vi "Check Watchdogs.vi"(7 "Check Period (ms)":u32=100, 8 "error in (no error)":errorcluster, 11 "RT - Analysis Data in in in in":T1={"Accel Sensistivity"=[0.0, 0.0, 0.0], "Cutoff Frequncies"=[{"LP Passband"=0.0, "HP Stopband"=0.0, "LP Stopband"=0.0, "HP Passband"=0.0}, {"LP Passband"=0.0, "HP Stopband"=0.0, "LP Stopband"=0.0, "HP Passband"=0.0}, {"LP Passband"=0.0, "HP Stopband"=0.0, "LP Stopband"=0.0, "HP Passband"=0.0}], "APU Setup File"={"Sensor Info"=[], "Calibration Info"=[], "CMM Table 106"=[], "CMM Table 106B "=[], "Accel Config"=[], "Report Sheet 1"=[], "Report Sheet 2"=[], "Report Sheet 3"=[]}, "RepairLevel"=""} {"Cutoff Frequncies"."HP Passband" min=1.0 step=1.0 format="%#.4f"; "Cutoff Frequncies"."LP Stopband" min=1.0 step=1.0 format="%#.4f"; "Cutoff Frequncies"."HP Stopband" min=1.0 step=1.0 format="%#.4f"; "Cutoff Frequncies"."LP Passband" min=1.0 step=1.0 format="%#.4f"}) -> (0 "error out":errorcluster, 3 "RT - Analysis Data in in out":T1 {"Cutoff Frequncies"."HP Passband" min=1.0 step=1.0 format="%#.4f"; "Cutoff Frequncies"."LP Stopband" min=1.0 step=1.0 format="%#.4f"; "Cutoff Frequncies"."HP Stopband" min=1.0 step=1.0 format="%#.4f"; "Cutoff Frequncies"."LP Passband" min=1.0 step=1.0 format="%#.4f"})   [LabVIEW 2018, in "RT - Analysis.lvlib"]
doc: "Runs through each Watchdog setting and checks for triggers.\n\n<b>Timer - Change Sample Rate</b>\nDBL0 : Timer Length\nDBL1 : New Sample Ratea\n\n<b>RPM Thresh - Insert Other</b> (Inserts Watchdog from variant)\nBool0 : T/F : RPMGreaterThan/RPMLessThan\nDBL0 : RPM Thresh Val\nVariant : Watchdog Cluster\n\n<b>RPM Thresh - Check POPD</b>\nBool0 : T/F : RPMGreaterThan/RPMLessThan\nBool1 : T/F : POPDGreaterThan/POPDLessThan\nDBL0 : RPM Thresh Val\nDBL1 : POPD Thresh Val\n\n<b>RPM Thresh - StartStop Logging</b>\nBool0 : T/F : RPMGreaterThan/RPMLessThan\nBool1 : T/F : StartLogg/FalseLogg\nDBL0 : Thresh Val"
uses:
  RT - Analysis.lvlib
  RT - Host Comms/RT - Host Comms.lvlib
  Public Controls/Alert Data.ctl
  Private Controls/Watchdog Settings.ctl
  Private Controls/RT-Analysis Data.ctl
  Modules/Testing UI 3/Private Controls/Cutoff Frequency.ctl
  Modules/Testing UI 3/Testing UI 3.lvlib
  Top Level/Shared Controls/APU Setup File.ctl
panel:
  # "Highpass Cutoff Frequency"
  # "Lowpass Cutoff Frequency"
  # "Highpass Cutoff Frequency"
  # "Lowpass Cutoff Frequency"
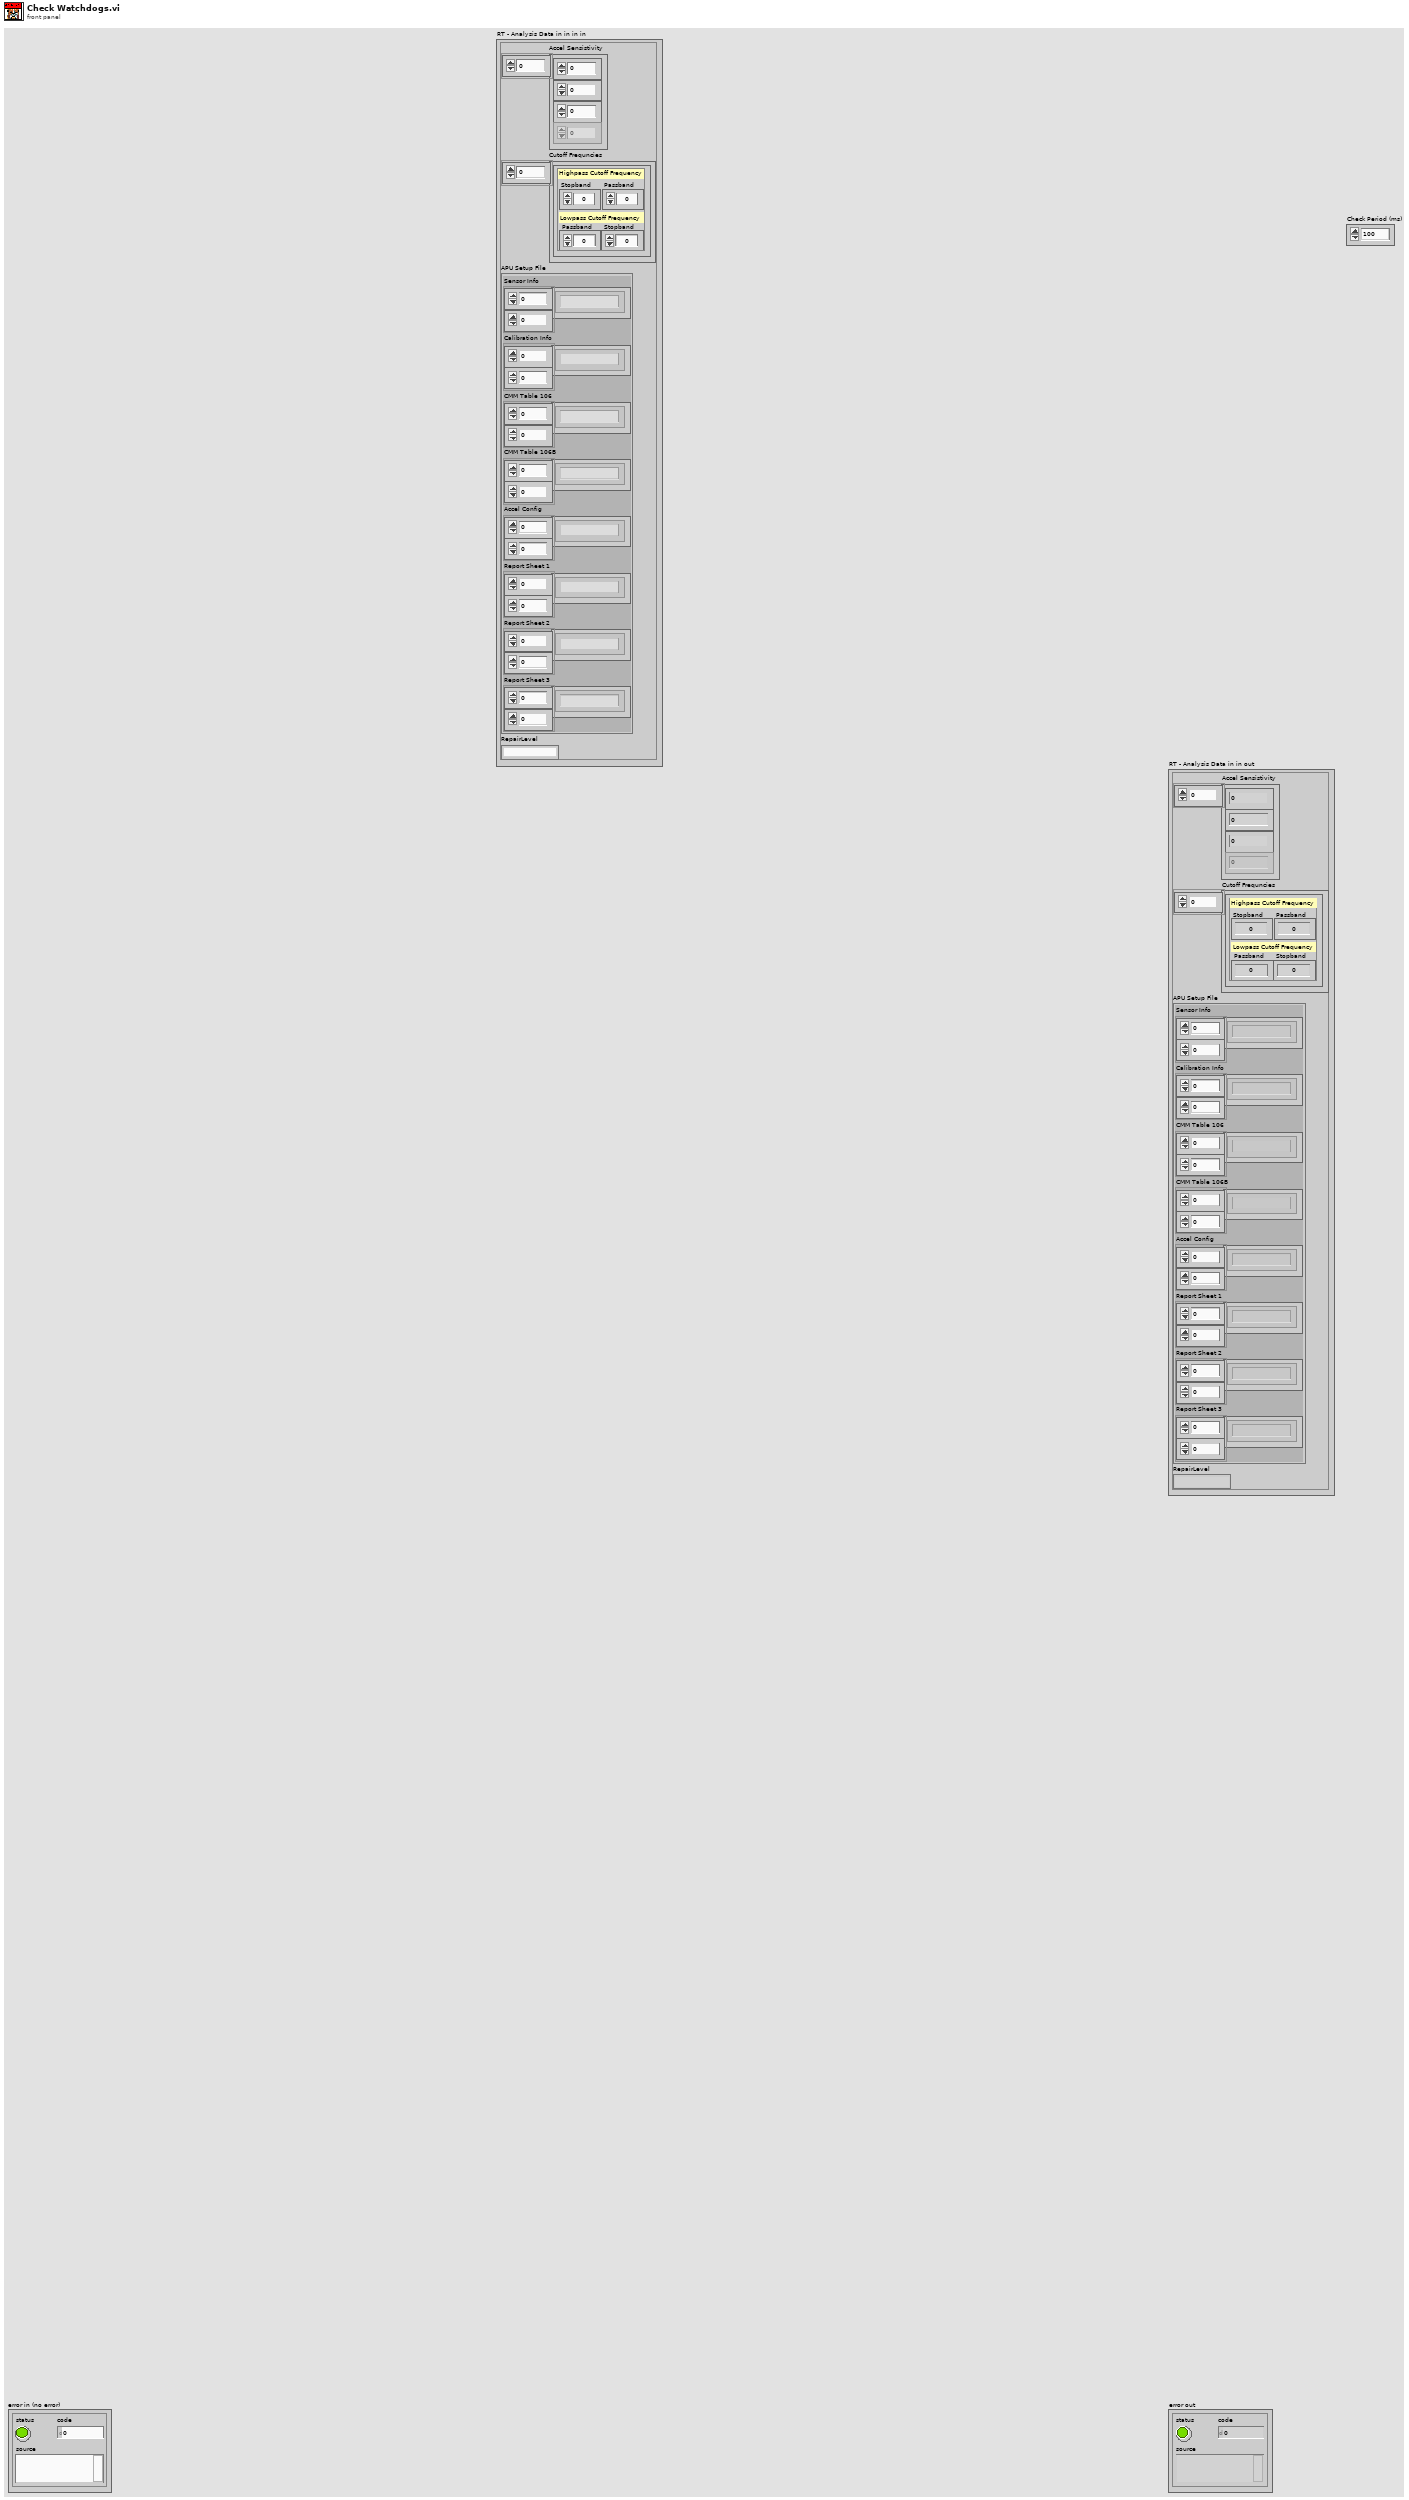
[diagram p1: front panel]
types:
  T1 = typedef "RT - Analysis.lvlib/RT-Analysis Data.ctl" = cluster{"Accel Sensistivity":dbl[], "Cutoff Frequncies":T2[], "APU Setup File":T3, "RepairLevel":string}
  T2 = typedef "Testing UI 3.lvlib/Cutoff Frequency.ctl" = cluster{"LP Passband":dbl, "HP Stopband":dbl, "LP Stopband":dbl, "HP Passband":dbl}
  T3 = typedef "APU Setup File.ctl" = cluster{"Sensor Info":string[][], "Calibration Info":string[][], "CMM Table 106":string[][], "CMM Table 106B ":string[][], "Accel Config":string[][], "Report Sheet 1":string[][], "Report Sheet 2":string[][], "Report Sheet 3":string[][]}
  T4 = typedef "RT - Analysis.lvlib/Watchdog Settings.ctl" = cluster{"Watchdog Action":enum16{"Disabled", "Timer - Change Sample Rate", "RPM Thresh - Insert Other", "RPM Thresh - Check POPD", "RPM Thresh - StartStop Logging"}, "Timer Start":timestamp, "[Watchdog Bools]":bool[], "[Watchdog DBLs]":dbl[], "Watchdog Variant":variant}
  T5 = typedef "RT - Analysis.lvlib/Alert Data.ctl" = cluster{"Tag":string, "Value":dbl, "Alerts":bool[], "Thresh Val":dbl, "Thresh Len":dbl, "Thresh Type":enum16{"Neither", "Max", "Min"}}
  T6 = enum16{"Disabled", "Timer - Change Sample Rate", "RPM Thresh - Insert Other", "RPM Thresh - Check POPD", "RPM Thresh - StartStop Logging"}
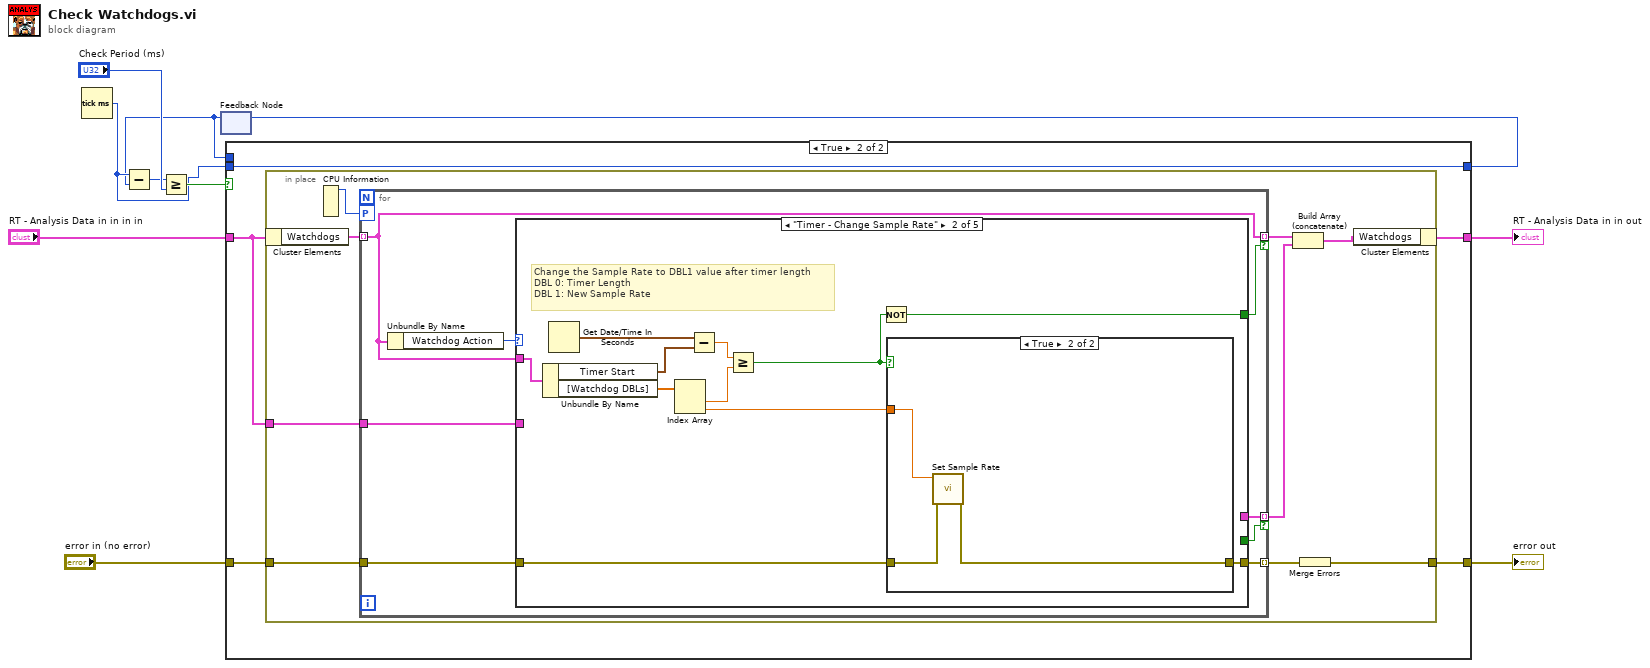
[diagram p0: block diagram]
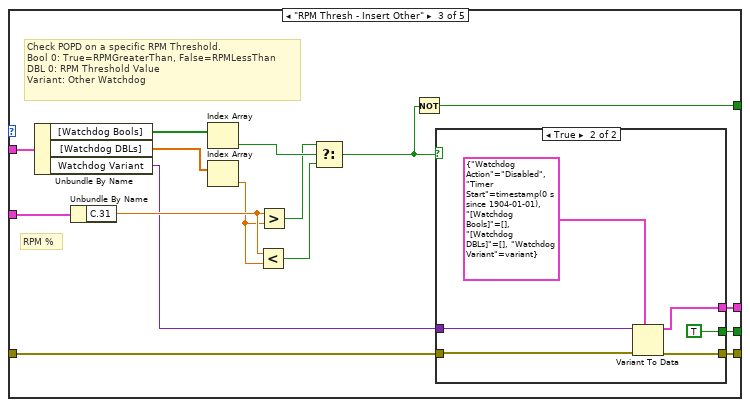
[diagram p5: hidden frame]
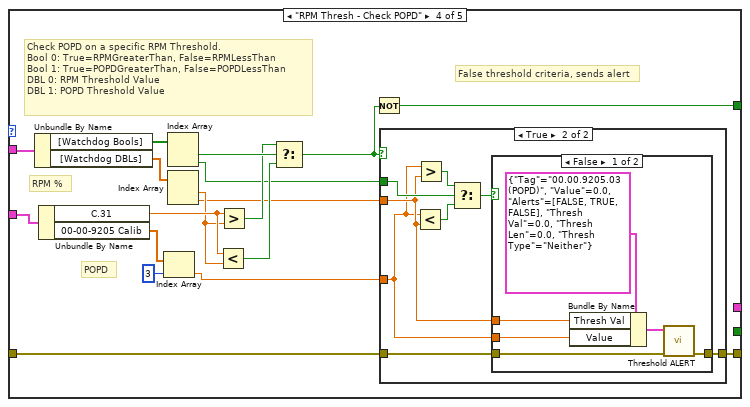
[diagram p7: hidden frame]
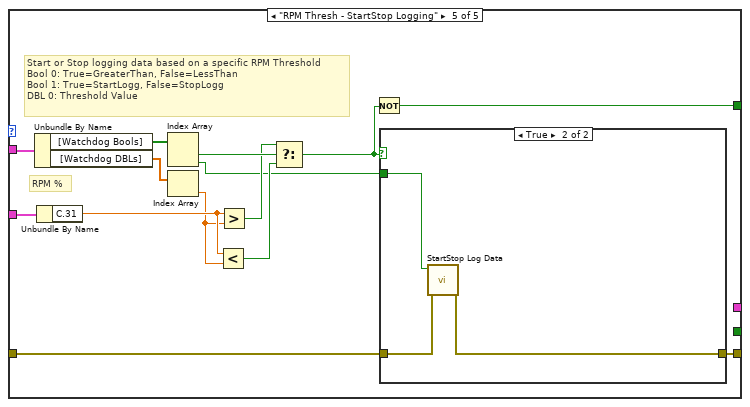
[diagram p10: hidden frame]
diagram:
  n1 = Tick Count (ms)() -> (millisecond timer value=w2:u32)
  n2 = feedback #1() -> (w1:u32)  [unwired: 1 in]
  n3 = Subtract(x=w2, y=w1) -> (x-y=w5:u32)
  n4 = Greater Or Equal?(x=w5, y="Check Period (ms)") -> (x >= y?=w4:bool)
  n5 = case shown="True" w4 {
    tunnel: [w11 w18] -> w10
    tunnel: [w12 w17] -> w9
    tunnel: "RT - Analysis Data in in in in" -> [w12 w16]
    tunnel: "error in (no error)" -> [w11 w15]
    tunnel: [w13 w14] -> w3
    tunnel: w2 -> [_ w14]
    tunnel: w1 -> [w13 _]
    frame False {
    }
    frame True {
      n6 = in-place {
        in-place-border: w15 -> [w27]
        in-place-border: w16 -> [w26]
        in-place-border: [w22] -> w18
        n7 = in-place-cluster #2(w16) -> ("Watchdogs"=w25:T4[])
        n8 = CPU Information() -> (4:w21:i32)  [unwired: 3 out]
        n9 = for {
          tunnel: w26 -> [w34]
          tunnel: w25 -> [w33] mode=indexing
          tunnel: [w33] -> w24 mode=indexing if=w32
          tunnel: w27 -> [w31]
          tunnel: [w30] -> w23 mode=indexing
          workers-P: w21 -> [_]
          tunnel: [w29] -> w19 mode=indexing if=w28
          n10 = Unbundle By Name(w33) -> ("Watchdog Action"=w35:T6)
          n11 = case shown="\"Timer - Change Sample Rate\"" w35 {
            tunnel: w33 -> [_ w47 w67 w92 w122]
            tunnel: w34 -> [_ _ w63 w88 w118]
            tunnel: [_ w45 w57 w82 w112] -> w32
            tunnel: w31 -> [w36 w44 w56 w81 w111]
            tunnel: [w36 w43 w55 w80 w110] -> w30
            tunnel: [_ _ w53 _ _] -> w29
            tunnel: [_ _ w52 _ _] -> w28
            frame "Disabled", Default {
              # "Don't keep this watchdog"
            }
            frame "Timer - Change Sample Rate" {
              # "Change the Sample Rate to DBL1 value after timer length\nDBL 0: Timer Length\nDBL 1: New Sample Rate"
              n12 = Unbundle By Name(w47) -> ("Timer Start"=w41:timestamp, "[Watchdog DBLs]"=w46:dbl[])
              n13 = Get Date/Time In Seconds() -> (seconds since 1Jan1904=w42:timestamp)
              n14 = Index Array(array=w46) -> (element #1=w39:dbl, element #2=w37:dbl)  [unwired: 2 in]
              n15 = Subtract(x=w42, y=w41) -> (x-y=w40:dbl)
              n16 = Greater Or Equal?(x=w40, y=w39) -> (x >= y?=w38:bool)
              n17 = Not(x=w38) -> (.not. x?=w45:bool)
              n18 = case shown="True" w38 {
                tunnel: w37 -> [_ w49]
                tunnel: w44 -> [w48 w51]
                tunnel: [w48 w50] -> w43
                frame False {
                }
                frame True {
                  n19 = call "Set Sample Rate.vi"("error in (no error)"=w51, "Sample Rate"=w49) -> ("error out"=w50:errorcluster)  [unwired: 9 in]
                }
              }
            }
            frame "RPM Thresh - Insert Other" {
              # "RPM %"
              # "Check POPD on a specific RPM Threshold.\nBool 0: True=RPMGreaterThan, False=RPMLessThan\nDBL 0: RPM Threshold Value\nVariant: Other Watchdog"
              n20 = Unbundle By Name(w67) -> ("[Watchdog Bools]"=w66:bool[], "[Watchdog DBLs]"=w65:dbl[], "Watchdog Variant"=w54:variant)
              n21 = Unbundle By Name(w63) -> ("C.31"=w62:dbl)
              n22 = Index Array(array=w66) -> (element=w64:bool)  [unwired: 1 in]
              n23 = Index Array(array=w65) -> (element=w61:dbl)  [unwired: 1 in]
              n24 = Less?(x=w62, y=w61) -> (x < y?=w59:bool)
              n25 = Greater?(x=w62, y=w61) -> (0:w60:bool)
              n26 = Select(t=w60, s=w64, f=w59) -> (s? t:f=w58:bool)
              n27 = Not(x=w58) -> (.not. x?=w57:bool)
              n28 = case shown="True" w58 {
                tunnel: w56 -> [w68 w74]
                tunnel: [w68 w70] -> w55
                tunnel: w54 -> [_ w73]
                tunnel: [_ w72] -> w53
                tunnel: [_ TRUE] -> w52
                frame False {
                }
                frame True {
                  n29 = Variant To Data(error in=w74, type=T4 {"Watchdog Action"=enum."Disabled", "Timer Start"=timestamp(0 s since 1904-01-01), "[Watchdog Bools]"=[], "[Watchdog DBLs]"=[], "Watchdog Variant"=variant} ("Watchdog Setting"), Variant=w73) -> (data=w72:T4, error out=w70:errorcluster)
                }
              }
            }
            frame "RPM Thresh - Check POPD" {
              # "False threshold criteria, sends alert"
              # "POPD"
              # "RPM %"
              # "Check POPD on a specific RPM Threshold.\nBool 0: True=RPMGreaterThan, False=RPMLessThan\nBool 1: True=POPDGreaterThan, False=POPDLessThan\nDBL 0: RPM Threshold Value\nDBL 1: POPD Threshold Value"
              n30 = Unbundle By Name(w92) -> ("[Watchdog Bools]"=w91:bool[], "[Watchdog DBLs]"=w90:dbl[])
              n31 = Unbundle By Name(w88) -> ("C.31"=w87:dbl, "00-00-9205 Calib"=w78:dbl[])
              n32 = Index Array(array=w78, index=3) -> (element=w76:dbl)
              n33 = Index Array(array=w91) -> (element #1=w89:bool, element #2=w79:bool)  [unwired: 2 in]
              n34 = Index Array(array=w90) -> (element #1=w86:dbl, element #2=w75:dbl)  [unwired: 2 in]
              n35 = Less?(x=w87, y=w86) -> (x < y?=w84:bool)
              n36 = Greater?(x=w87, y=w86) -> (0:w85:bool)
              n37 = Select(t=w85, s=w89, f=w84) -> (s? t:f=w83:bool)
              n38 = Not(x=w83) -> (.not. x?=w82:bool)
              n39 = case shown="True" w83 {
                tunnel: w79 -> [_ w101]
                tunnel: w81 -> [w93 w97]
                tunnel: [w93 w96] -> w80
                tunnel: w76 -> [_ w94]
                tunnel: w75 -> [_ w95]
                frame False {
                }
                frame True {
                  n40 = Less?(x=w94, y=w95) -> (x < y?=w99:bool)
                  n41 = Greater?(x=w94, y=w95) -> (0:w100:bool)
                  n42 = Select(t=w100, s=w101, f=w99) -> (s? t:f=w98:bool)
                  n43 = case shown="False" w98 {
                    tunnel: w97 -> [w105 w108]
                    tunnel: [w104 w108] -> w96
                    tunnel: w95 -> [w103 _]
                    tunnel: w94 -> [w102 _]
                    frame False {
                      n44 = Bundle By Name(cluster=T5 {"Tag"="00.00.9205.03 (POPD)", "Value"=0.0, "Alerts"=[FALSE, TRUE, FALSE], "Thresh Val"=0.0, "Thresh Len"=0.0, "Thresh Type"=enum."Neither"} ("Alert Data"), "Thresh Val"=w103, "Value"=w102) -> (w106:T5)
                      n45 = call "Threshold ALERT.vi"("error in (no error)"=w105, "Alert Data"=w106) -> ("error out"=w104:errorcluster)  [unwired: 9 in]
                    }
                    frame True {
                    }
                  }
                }
              }
            }
            frame "RPM Thresh - StartStop Logging" {
              # "RPM %"
              # "Start or Stop logging data based on a specific RPM Threshold\nBool 0: True=GreaterThan, False=LessThan\nBool 1: True=StartLogg, False=StopLogg\nDBL 0: Threshold Value"
              n46 = Unbundle By Name(w122) -> ("[Watchdog Bools]"=w121:bool[], "[Watchdog DBLs]"=w120:dbl[])
              n47 = Unbundle By Name(w118) -> ("C.31"=w117:dbl)
              n48 = Index Array(array=w121) -> (element #1=w119:bool, element #2=w109:bool)  [unwired: 2 in]
              n49 = Index Array(array=w120) -> (element=w116:dbl)  [unwired: 1 in]
              n50 = Less?(x=w117, y=w116) -> (x < y?=w114:bool)
              n51 = Greater?(x=w117, y=w116) -> (0:w115:bool)
              n52 = Select(t=w115, s=w119, f=w114) -> (s? t:f=w113:bool)
              n53 = Not(x=w113) -> (.not. x?=w112:bool)
              n54 = case shown="True" w113 {
                tunnel: w109 -> [_ w124]
                tunnel: w111 -> [w123 w126]
                tunnel: [w123 w125] -> w110
                frame False {
                }
                frame True {
                  n55 = call "StartStop Log Data.vi"("error in (no error)"=w126, "Start/Stop (F:Stop)"=w124) -> ("error out"=w125:errorcluster)  [unwired: 9 in]
                }
              }
            }
          }
        }
        n56 = Build Array (concatenate)(w24, w19) -> (w20:T4[])
        n57 = Merge Errors(w23) -> (w22:errorcluster)
        n58 = in-place-cluster #2("Watchdogs"=w20) -> (w17:T1)
      }
    }
  }
  "error out" <- w10
  "RT - Analysis Data in in out" <- w9
  n59 = feedback-in #1(w3) -> ()
